vi "Conversion tension température.vi"(11 "Data In":dbl[](array[numeric])) -> ()   [LabVIEW 2018]
panel:
  out "Data Out":dbl[](array[numeric])
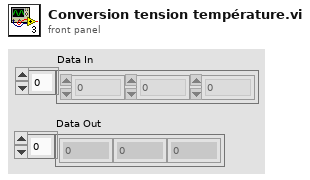
[diagram p1: front panel]
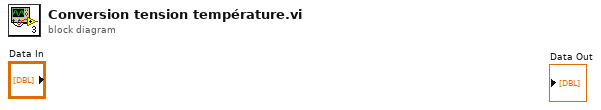
[diagram p0: block diagram]
diagram:
